vi "dfd_FXP PtByPt Direct IIR I.vi"(0 "x":T7={"value"=0, "wl"=0, "iwl"=0, "Signed"=TRUE} {"value" format="%.0x"}, 1 "coef b[0..M]":T6, 2 "coef a[1..N]":T6, 4 "yState tmp in":i64[](array[numeric]), 5 "filtering statistics in":T5(array[cluster]) {"statistics information"."min value" format="%.2f"; "statistics information"."max value" format="%.2f"; "Quantizer Source" items=["Coefficients a/k"=0, "Coefficients b/v"=7, "Input"=1, "Output"=2, "Multiplicand"=3, "Product"=4, "Sum"=5, "Delay"=6]}, 6 "FXPOPs":T1[](array[typedef]) {"source" items=["Coef a/k"=0, "Coef b/v"=7, "Input"=1, "Output"=2, "Multiplicand"=3, "Product"=4, "Sum"=5, "Delay"=6, "Gain"=8]}, 7 "xState in":i64[](array[numeric]), 9 "yState in":i64[](array[numeric])) -> (11 "yState out":i64[](array[numeric]), 13 "xState out":i64[](array[numeric]), 14 "filtered x":T7={"value"=0, "wl"=0, "iwl"=0, "Signed"=TRUE} {"value" format="%.0x"}, 18 "yState tmp out":i64[](array[numeric]), 19 "filtering statistics out":T5(array[cluster]) {"statistics information"."min value" format="%.2f"; "statistics information"."max value" format="%.2f"; "Quantizer Source" items=["Coefficients a/k"=0, "Coefficients b/v"=7, "Input"=1, "Output"=2, "Multiplicand"=3, "Product"=4, "Sum"=5, "Delay"=6]})   [LabVIEW 2017, in "NI_DigFilter_FXP.lvlib"]
uses:
  <vilib>/addons/Digital Filter Design/NI_DigFilter_FXP.lvlib
  <vilib>/addons/Digital Filter Design/_Objects.llb/dfd_DFXP Data Type (scaler).ctl
  <vilib>/addons/Digital Filter Design/_Objects.llb/dfd_DFXP Data Type (vector).ctl
  <vilib>/addons/Digital Filter Design/_Objects.llb/DFD Quantization Sources.ctl
  <vilib>/addons/Digital Filter Design/_Objects.llb/DFD FXP Statistics Data.ctl
  <vilib>/addons/Digital Filter Design/_Objects.llb/dfd_DFXP Operation Parameter.ctl
  <vilib>/addons/Digital Filter Design/_Objects.llb/dfd_Internal Quantization Srcs.ctl
  <vilib>/addons/Digital Filter Design/NI_DigFilterLicensed.lvlib
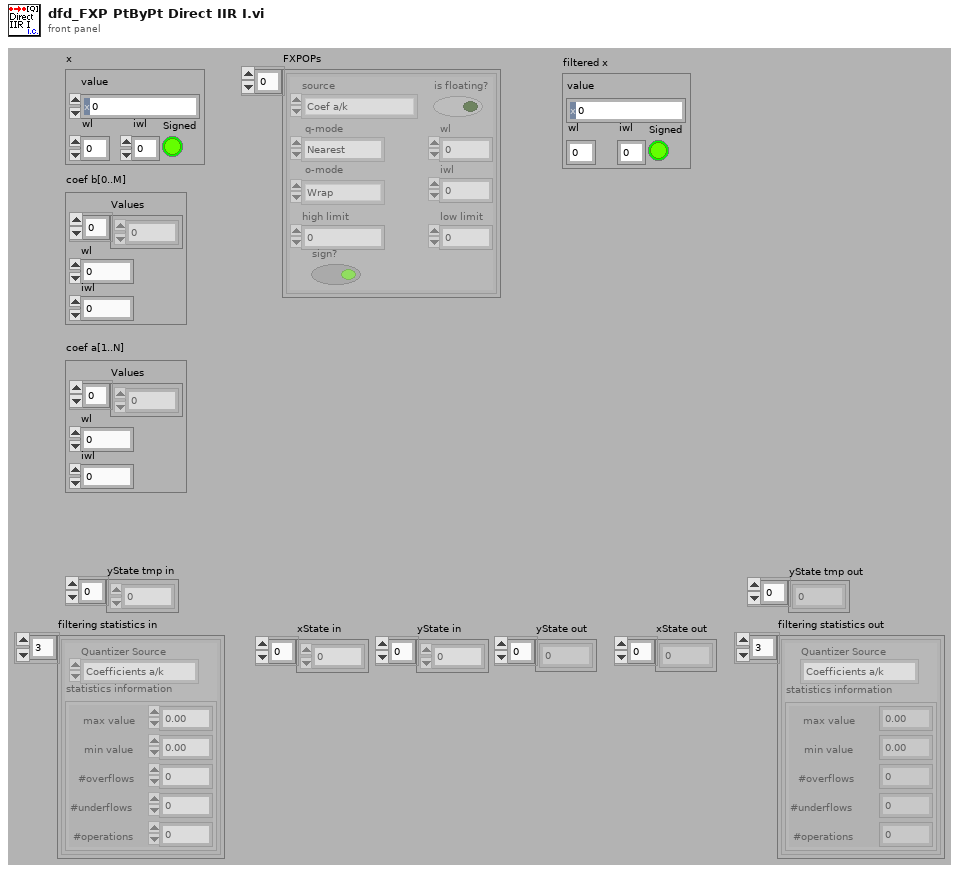
[diagram p1: front panel]
types:
  T1 = typedef "dfd_DFXP Operation Parameter.ctl" = cluster{"source":T2, "is floating?":bool, "o-mode":enum16{"Saturation", "Wrap"}, "q-mode":enum16{"Nearest", "Truncation"}, "wl":i16, "high limit":i64, "low limit":i64, "iwl":i16, "sign?":bool}
  T2 = typedef "NI_DigFilterLicensed.lvlib/dfd_Internal Quantization Srcs.ctl" = u16
  T3 = typedef "NI_DigFilterLicensed.lvlib/DFD Quantization Sources.ctl" = u16
  T4 = typedef "NI_DigFilterLicensed.lvlib/DFD FXP Statistics Data.ctl" = cluster{"max value":ext, "min value":ext, "#overflows":i32, "#underflows":i32, "#operations":i32}
  T5 = cluster{"Quantizer Source":T3, "statistics information":T4}[]
  T6 = typedef "dfd_DFXP Data Type (vector).ctl" = cluster{"Values":i64[], "wl":i16, "iwl":i16}
  T7 = typedef "dfd_DFXP Data Type (scaler).ctl" = cluster{"value":i64, "wl":i16, "iwl":i16, "Signed":bool}
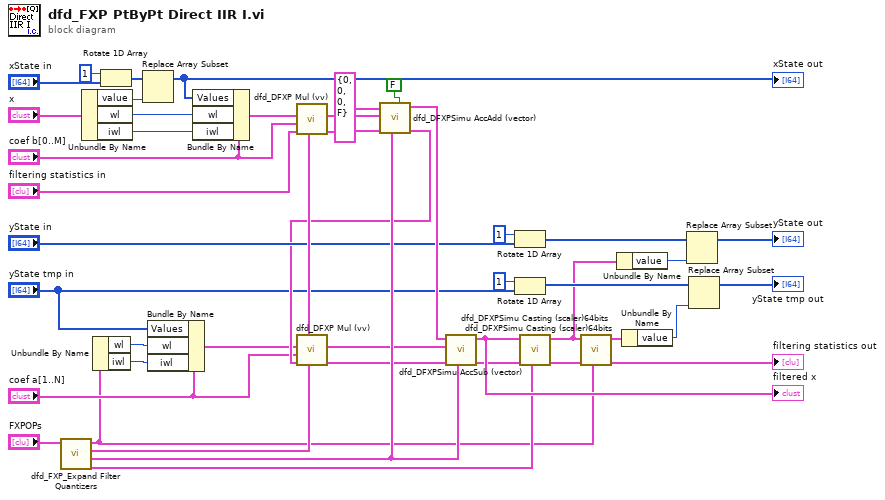
[diagram p0: block diagram]
diagram:
  n1 = call <vilib>:"dfd_FXP_Expand Filter Quantizers.vi"("FXPOPs"="FXPOPs") -> ("Delay"=w39:T1, "Sum"=w43:T1, "Product"=w42:T1, "Multiplicand"=w6:T1)  [unwired: 7 out]
  n2 = Unbundle By Name("x") -> ("value"=w23:i64, "wl"=w19:i16, "iwl"=w18:i16)
  n3 = Unbundle By Name(w6) -> ("wl"=w14:i16, "iwl"=w13:i16)
  n4 = Rotate 1D Array(1:"xState in", 2:1 ("n")) -> (0:w37:i64[])
  n5 = Replace Array Subset(array=w37, new element=w23) -> (w40:i64[])  [unwired: 1 in]
  "xState out" <- w40
  n6 = Bundle By Name(cluster="coef a[1..N]", "Values"="yState tmp in", "wl"=w14, "iwl"=w13) -> (w12:T6)
  n7 = Bundle By Name(cluster="coef b[0..M]", "Values"=w40, "wl"=w19, "iwl"=w18) -> (w22:T6)
  n8 = call <vilib>:"dfd_DFXP Mul (vv).vi"("op params"=w42, "filtering statistics in"="filtering statistics in", "Value in 2"="coef b[0..M]", "Value in"=w22) -> ("filtering statistics out"=w33:T5, "Value out"=w34:T6)  [unwired: 6 out]
  n9 = call <vilib>:"dfd_DFXPSimu AccAdd (vector).vi"("quantize output?"=FALSE, "op params"=w43, "filtering statistics in"=w33, "addends"=w34, "acc in"=T7 {"value"=0, "wl"=0, "iwl"=0, "Signed"=FALSE}) -> ("filtering statistics out"=w16:T5, "acc out"=w31:T7)  [unwired: 5 out]
  n10 = call <vilib>:"dfd_DFXP Mul (vv).vi"("op params"=w42, "filtering statistics in"=w16, "Value in 2"="coef a[1..N]", "Value in"=w12) -> ("filtering statistics out"=w32:T5, "Value out"=w21:T6)  [unwired: 6 out]
  n11 = call <vilib>:"dfd_DFXPSimu AccSub (vector).vi"("op params"=w43, "filtering statistics in"=w32, "addends"=w21, "acc in"=w31) -> ("filtering statistics out"=w30:T5, "acc out"=w44:T7)  [unwired: 1 in, 5 out]
  "filtered x" <- w44
  n12 = Rotate 1D Array(1:"yState in", 2:1 ("n")) -> (0:w35:i64[])
  n13 = Rotate 1D Array(1:"yState tmp in", 2:1 ("n")) -> (0:w11:i64[])
  n14 = call <vilib>:"dfd_DFXPSimu Casting (scaler)64bits.vi"("op params"=w39, "filtering statistics in"=w30, "Value in"=w44) -> ("filtering statistics out"=w7:T5, "Value out"=w8:T7)  [unwired: 2 in, 5 out]
  n15 = call <vilib>:"dfd_DFXPSimu Casting (scaler)64bits.vi"("op params"=w6, "filtering statistics in"=w7, "Value in"=w8) -> ("filtering statistics out"=→"filtering statistics out":T5, "Value out"=w5:T7)  [unwired: 1 in, 6 out]
  n16 = Unbundle By Name(w8) -> ("value"=w20:i64)
  n17 = Unbundle By Name(w5) -> ("value"=w4:i64)
  n18 = Replace Array Subset(array=w35, new element=w20) -> (→"yState out":i64[])  [unwired: 1 in]
  n19 = Replace Array Subset(array=w11, new element=w4) -> (→"yState tmp out":i64[])  [unwired: 1 in]
